vi "Revision Query.vi"(8 "error in (no error)":errorcluster, 11 "VISA resource name":refnum<visa-resource-name>) -> (0 "error out":errorcluster, 1 "Instrument Firmware Revision":string, 2 "Instrument Driver Revision":string, 3 "VISA resource name out":refnum<visa-resource-name>)   [LabVIEW 2026, in "Agilent 33XXX Series.lvlib"]
doc: "This VI queries the current instrument firmware revision and instrument driver revision.\n\nFor detailed driver information including modification history, refer to the Readme file."
uses:
  Agilent 33XXX Series.lvlib
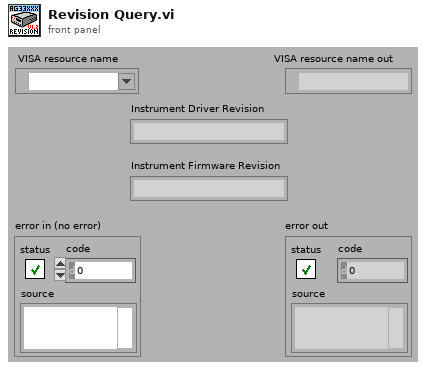
[diagram p1: front panel]
types:
  T1 = enum32{"invalid app kind", "Development System", "Run Time System", "Student Edition", "Embedded LabVIEW", "Evaluation", "Custom"}
  T2 = cluster{"Major":u16, "Minor":u16, "Fix":u16, "Build":u16}
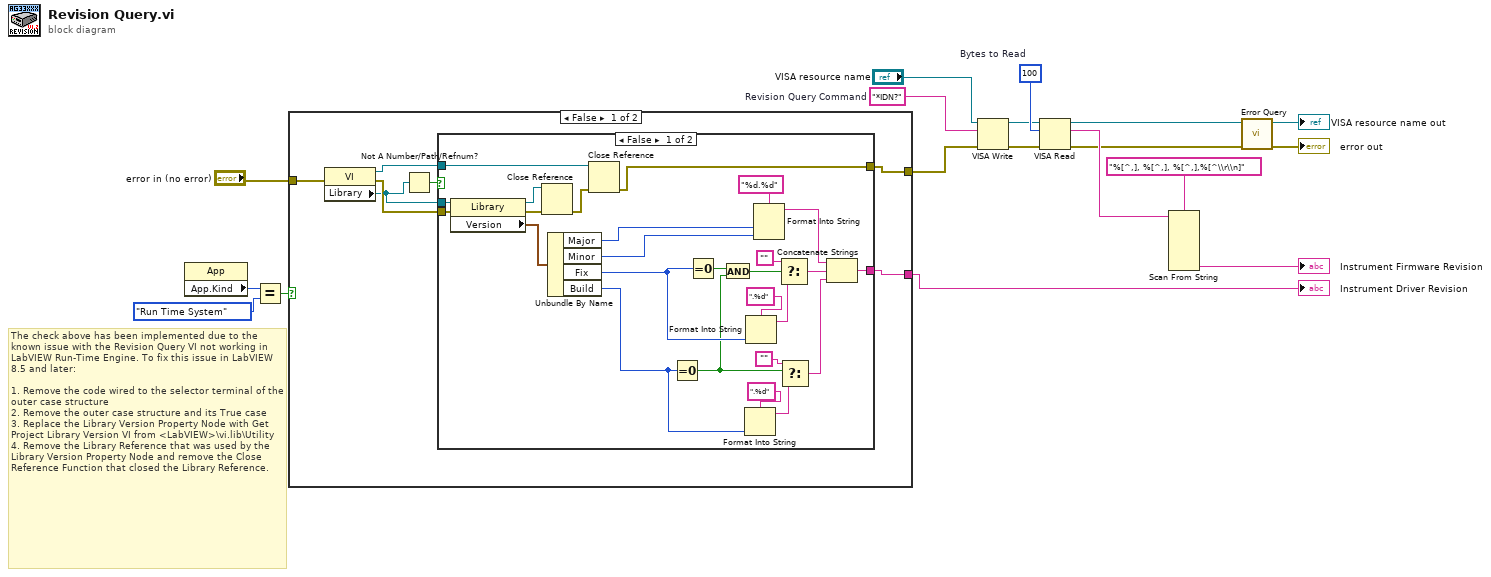
[diagram p0: block diagram]
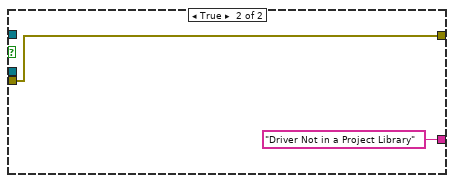
[diagram p2: hidden frame]
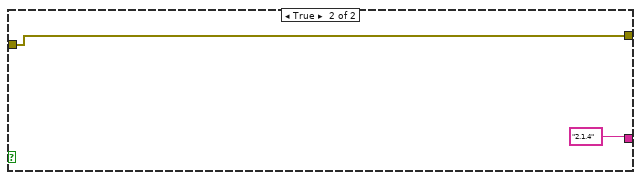
[diagram p3: hidden frame]
diagram:
  w13 = "*IDN?"  # Revision Query Command
  w16 = u32 100  # Bytes to Read
  # "The check above has been implemented due to the known issue with the Revision Query VI not working in LabVIEW Run-Time Engine. To fix this issue in LabVIEW 8.5 and later:\n\n1. Remove the code wired to the selector terminal of the outer case structure\n2. Remove the outer case structure and its True case\n3. Replace the Library Version Property Node with Get Project Library Version VI from <LabVIEW>\\vi.lib\\Utility\n4. Remove the Library Reference that was used by the Library Version Property Node and remove the Close Reference Function that closed the Library Reference."
  n1 = property class="App"() -> ("App.Kind"=w2:T1)  [unwired: 2 in, 2 out]
  n2 = Equal?(x=w2, y=T1."Run Time System") -> (x = y?=w3:bool)
  n3 = case shown="False" w3 {
    tunnel: "error in (no error)" -> [w25 w55]
    tunnel: [w20 "2.1.4"] -> w5
    tunnel: [w19 w55] -> w4
    frame False {
      n4 = property class="VI"(error in=w25) -> (reference out=w21:refnum<vi>, error out=w24:errorcluster, "Library"=w23:refnum<vi>)  [unwired: 1 in]
      n5 = Not A Number/Path/Refnum?(number/path/refnum=w23) -> (NaN/Path/Refnum?=w22:bool)
      n6 = case shown="False" w22 {
        tunnel: [w31 w52] -> w19
        tunnel: [w30 "Driver Not in a Project Library"] -> w20
        tunnel: w24 -> [w28 w52]
        tunnel: w23 -> [w27 _]
        tunnel: w21 -> [w26 _]
        frame False {
          n7 = property class="Library"(reference=w27, error in=w28) -> (reference out=w50:refnum<vi>, error out=w51:errorcluster, "Version"=w48:T2)
          n8 = Close Reference(reference=w50, error in (no error)=w51) -> (error out=w49:errorcluster)
          n9 = Unbundle By Name(w48) -> ("Major"=w38:u16, "Minor"=w37:u16, "Fix"=w35:u16, "Build"=w36:u16)
          n10 = Close Reference(reference=w26, error in (no error)=w49) -> (error out=w31:errorcluster)
          n11 = Equal To 0?(x=w36) -> (x = 0?=w33:bool)
          n12 = Equal To 0?(x=w35) -> (x = 0?=w34:bool)
          n13 = And(x=w34, y=w33) -> (x .and. y?=w32:bool)
          n14 = Format Into String(format string=".%d", w36) -> (resulting string=w41:string)  [unwired: 2 in, 1 out]
          n15 = Format Into String(format string=".%d", w35) -> (resulting string=w45:string)  [unwired: 2 in, 1 out]
          n16 = Format Into String(format string="%d.%d", w38, w37) -> (resulting string=w43:string)  [unwired: 2 in, 1 out]
          n17 = Select(t="", s=w32, f=w45) -> (s? t:f=w42:string)
          n18 = Select(t="", s=w33, f=w41) -> (s? t:f=w39:string)
          n19 = Concatenate Strings(w43, w42, w39) -> (w30:string)
        }
        frame True {
        }
      }
    }
    frame True {
    }
  }
  "Instrument Driver Revision" <- w5
  n20 = VISA Write(VISA resource name="VISA resource name", write buffer=w13, error in (no error)=w4) -> (VISA resource name out=w15:refnum<visa-resource-name>, error out=w14:errorcluster)  [unwired: 1 out]
  n21 = VISA Read(VISA resource name=w15, byte count=w16, error in (no error)=w14) -> (VISA resource name out=w9:refnum<visa-resource-name>, read buffer=w12:string, error out=w10:errorcluster)  [unwired: 1 out]
  n22 = Scan From String(format string="%[^,], %[^,], %[^,],%[^\\r\\n]", input string=w12) -> (output 4=→"Instrument Firmware Revision":string)  [unwired: 9 in, 3 out]
  n23 = call "Error Query.vi"("error in (no error)"=w10, "VISA resource name"=w9) -> ("error out"=→"error out":errorcluster, "VISA resource name out"=→"VISA resource name out":refnum<visa-resource-name>)  [unwired: 6 in, 2 out]
